vi "RP hub write.vi"(8 "Error In":errorcluster, 9 "hub port":u64=2, 10 "data in":string, 11 "connection ID":refnum<k5>) -> (0 "Error Out":errorcluster, 3 "connection ID out":refnum<k5>)   [LabVIEW 2024]
uses:
  RP Command.ctl
  RP Write Command TCP.vi
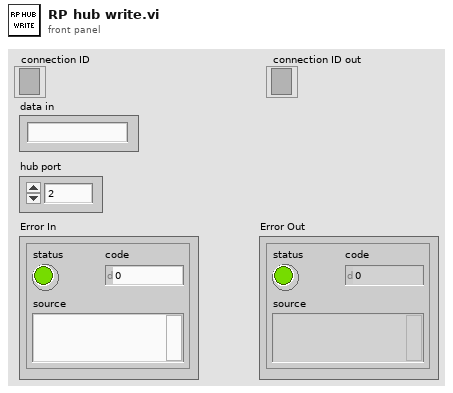
[diagram p1: front panel]
types:
  T1 = typedef "RP Command.ctl" = enum16{"Reset", "Read IDN", "Stop server", "Get status", "Get temperature", "Connect client", "Arm", "Software trigger", "Get whole buffer", "Get chunk", "System call", "Get config", "Set config", "Recieve data", "Recieve Calibartion", "Transmit data"}
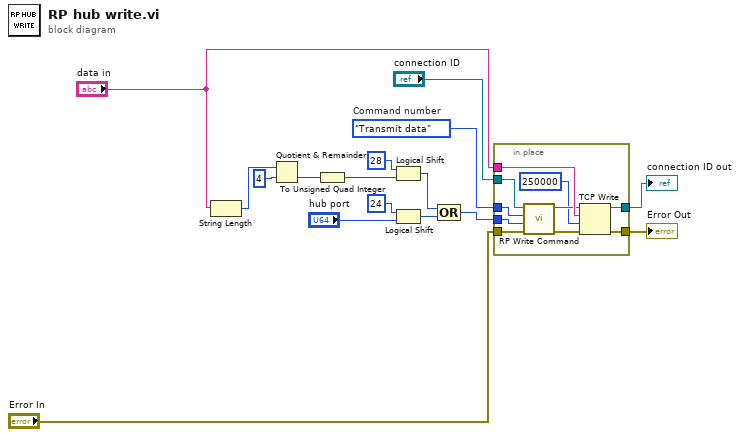
[diagram p0: block diagram]
diagram:
  w12 = RP_Command."Transmit data"  # Command number
  n1 = String Length(string="data in") -> (length=w11:i32)
  n2 = Quotient & Remainder(x=w11, y=4) -> (floor(x/y)=w7:i32)  [unwired: 1 out]
  n3 = To Unsigned Quad Integer(1:w7) -> (0:w3:u64)
  n4 = Logical Shift(y=i16 28, x=w3) -> (x << y=w5:u64)
  n5 = Logical Shift(y=i16 24, x="hub port") -> (x << y=w4:u64)
  n6 = Compound Arithmetic op=OR(w5, w4) -> (w2:u64)
  n7 = in-place {
    in-place-border: "connection ID" -> [w26]
    in-place-border: "data in" -> [w25]
    in-place-border: [w23] -> w15
    in-place-border: [w22] -> w14
    in-place-border: "Error In" -> [w21]
    in-place-border: w12 -> [w19]
    in-place-border: w2 -> [w18]
    n8 = call-poly "RP Write Command.vi"("Error In"=w21, "Command payload"=w18, "Command number"=w19, "connection ID"=w26) -> ("Error Out"=w20:errorcluster, "connection ID out"=w24:refnum<k5>)  [unwired: 4 in, 2 out]
    n9 = TCP Write(connection ID=w24, data in=w25, error in (no error)=w20, 9:250000 ("timeout ms (25000)")) -> (connection ID out=w22:refnum<k5>, error out=w23:errorcluster)  [unwired: 1 out]
  }
  "connection ID out" <- w14
  "Error Out" <- w15
